vi "trafficLight.vi"() -> ()   [LabVIEW 2019]
uses:
  TrafficLight/control/Control 1.ctl
panel:
  in  "stop 2":bool
  in  "Process Stop Button":bool
  in  "green sec":i32
  in  "yellow sec":i32
  in  "red sec":i32
  out "red":bool
  out "yellow":bool
  out "green":bool
  out "秒數積累":i32
  in  "快走速度(ms)":u32=100
  in  "慢走速度(ms)":u32=200
  in  "轉速時間(S)":dbl=5.0
  out "Array":bool[][](array[boolean])=[[FALSE, FALSE, FALSE, FALSE, FALSE, FALSE, FALSE, FALSE, FALSE, FALSE, FALSE, FALSE, FALSE, FALSE, FALSE], [FALSE, FALSE, FALSE, FALSE, FALSE, FALSE, TRUE, TRUE, FALSE, FALSE, FALSE, FALSE, FALSE, FALSE, FALSE], [FALSE, FALSE, FALSE, FALSE, FALSE, TRUE, TRUE, TRUE, TRUE, FALSE, FALSE, FALSE, FALSE, FALSE, FALSE], [FALSE, FALSE, FALSE, FALSE, FALSE, TRUE, TRUE, TRUE, TRUE, FALSE, FALSE, FALSE, FALSE, FALSE, FALSE], [FALSE, FALSE, FALSE, FALSE, FALSE, FALSE, TRUE, TRUE, FALSE, FALSE, FALSE, FALSE, FALSE, FALSE, FALSE], [FALSE, FALSE, FALSE, FALSE, TRUE, TRUE, TRUE, TRUE, TRUE, TRUE, FALSE, FALSE, FALSE, FALSE, FALSE], [FALSE, FALSE, FALSE, TRUE, TRUE, TRUE, TRUE, TRUE, TRUE, TRUE, TRUE, FALSE, FALSE, FALSE, FALSE], [FALSE, FALSE, TRUE, TRUE, FALSE, TRUE, TRUE, TRUE, TRUE, FALSE, TRUE, TRUE, FALSE, FALSE, FALSE], [FALSE, FALSE, TRUE, TRUE, FALSE, TRUE, TRUE, TRUE, TRUE, FALSE, TRUE, TRUE, FALSE, FALSE, FALSE], [FALSE, FALSE, TRUE, FALSE, FALSE, TRUE, TRUE, TRUE, TRUE, FALSE, FALSE, TRUE, FALSE, FALSE, FALSE], [FALSE, FALSE, FALSE, FALSE, FALSE, TRUE, TRUE, TRUE, TRUE, FALSE, FALSE, FALSE, FALSE, FALSE, FALSE], [FALSE, FALSE, FALSE, FALSE, TRUE, TRUE, FALSE, FALSE, TRUE, TRUE, FALSE, FALSE, FALSE, FALSE, FALSE], [FALSE, FALSE, FALSE, FALSE, TRUE, TRUE, FALSE, FALSE, TRUE, TRUE, FALSE, FALSE, FALSE, FALSE, FALSE], [FALSE, FALSE, FALSE, TRUE, TRUE, FALSE, FALSE, FALSE, FALSE, TRUE, TRUE, FALSE, FALSE, FALSE, FALSE], [FALSE, FALSE, FALSE, TRUE, TRUE, FALSE, FALSE, FALSE, FALSE, TRUE, TRUE, FALSE, FALSE, FALSE, FALSE], [FALSE, FALSE, FALSE, TRUE, TRUE, FALSE, FALSE, FALSE, FALSE, TRUE, TRUE, FALSE, FALSE, FALSE, FALSE], [FALSE, FALSE, FALSE, FALSE, FALSE, FALSE, FALSE, FALSE, FALSE, FALSE, FALSE, FALSE, FALSE, FALSE, FALSE]]
  out "subarray":bool[][](array[boolean])
  in  "x-1":dbl
  out "剩餘時間 2":u32
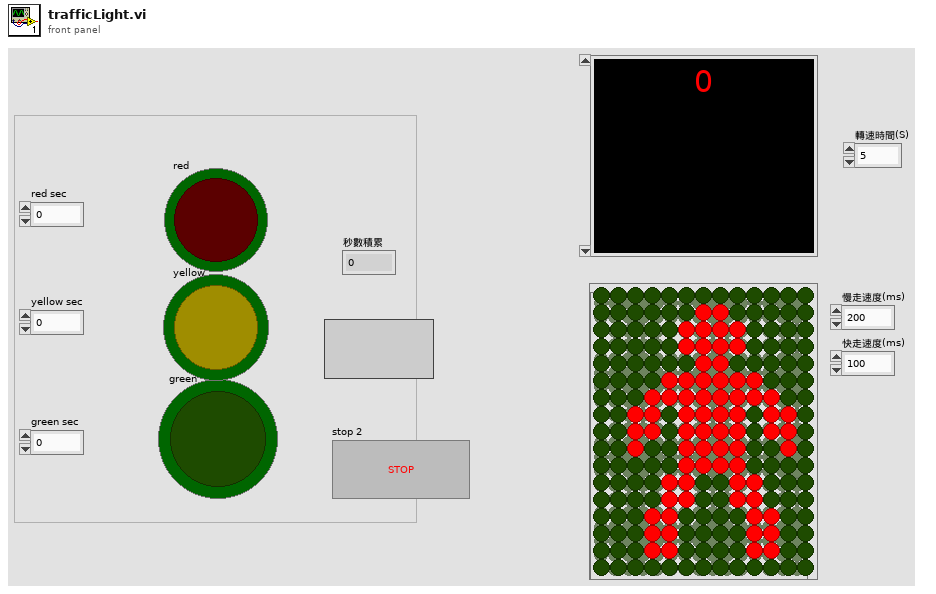
[diagram p1: front panel]
types:
  T1 = typedef "Control 1.ctl" = enum16{"red", "yellow", "green"}
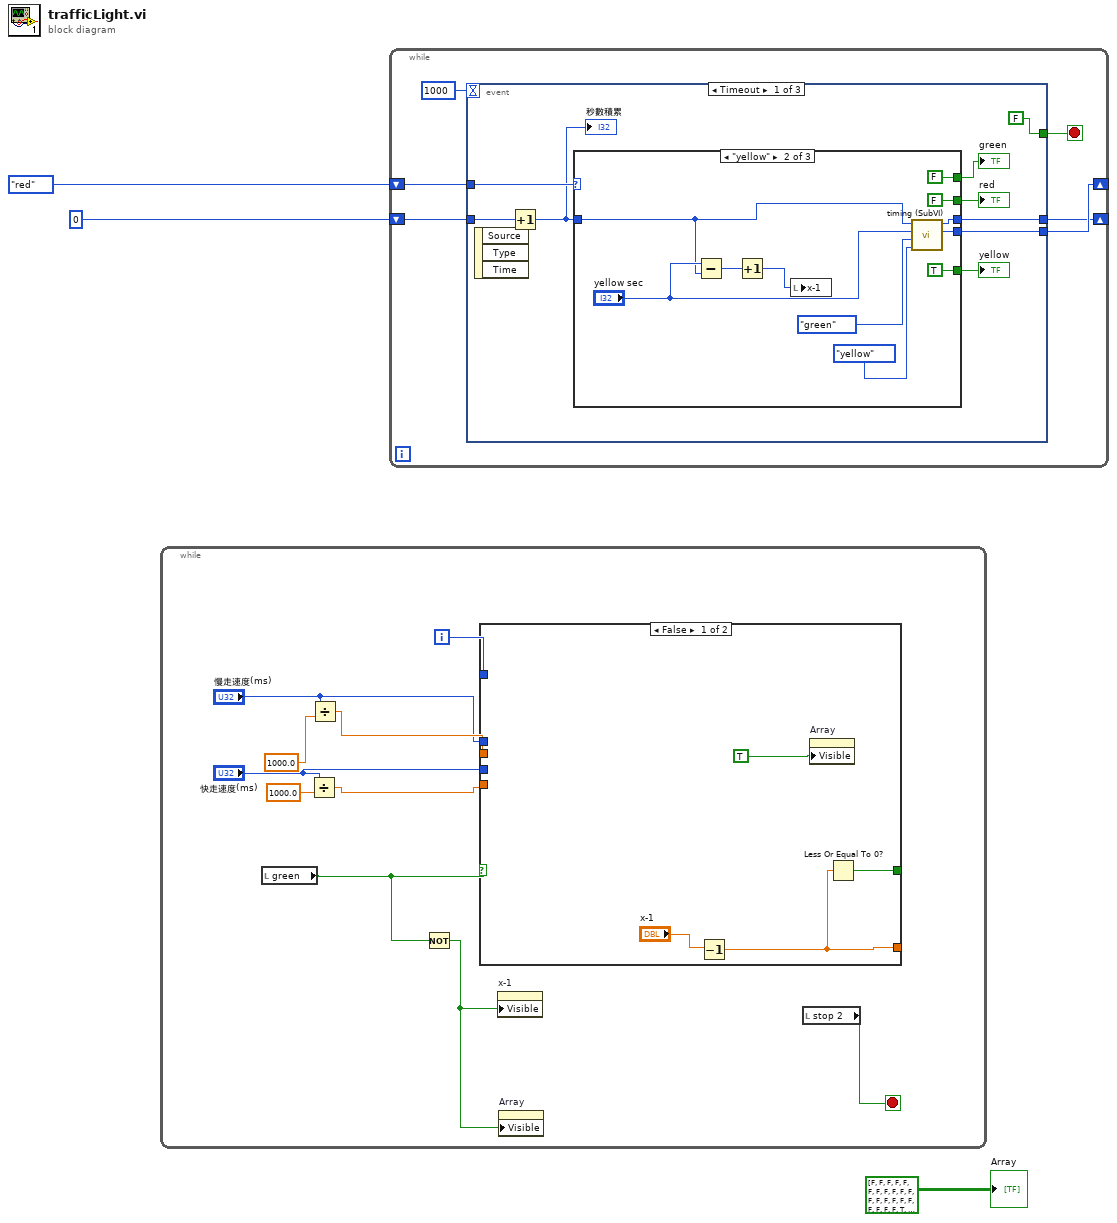
[diagram p0: block diagram]
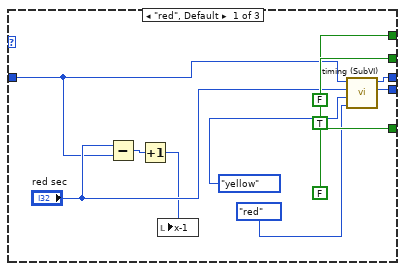
[diagram p2: hidden frame]
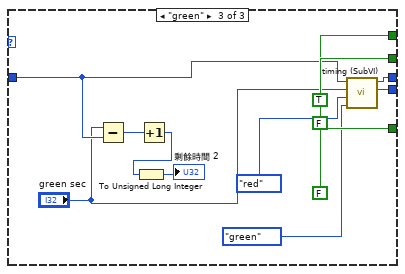
[diagram p3: hidden frame]
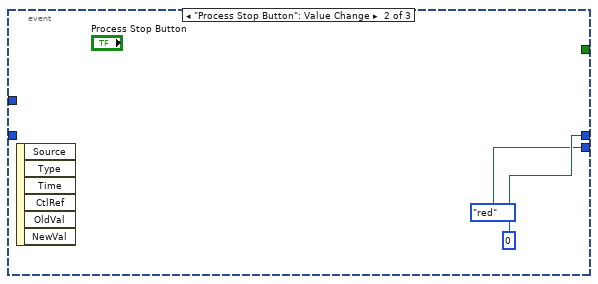
[diagram p4: hidden frame]
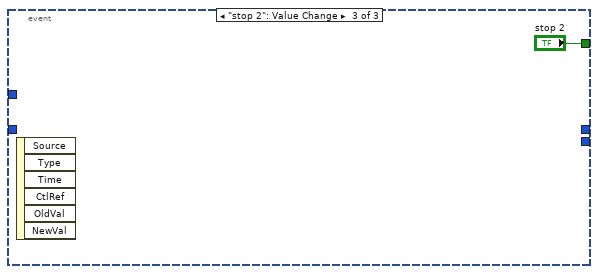
[diagram p5: hidden frame]
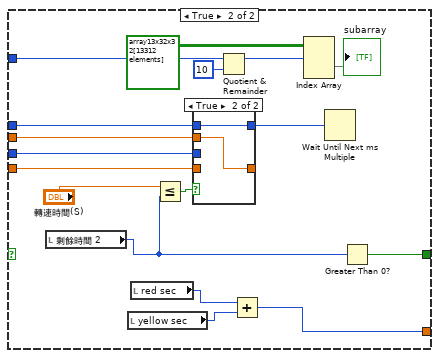
[diagram p6: hidden frame]
diagram:
  n1 = while {
    i -> [w12]
    stop <- w11 stop-if-true
    n2 = local read "green"() -> (w10:bool)
    n3 = Divide(x="快走速度(ms)", y=1000.0) -> (x/y=w6:dbl)
    n4 = Divide(x="慢走速度(ms)", y=1000.0) -> (x/y=w7:dbl)
    n5 = Not(x=w10) -> (.not. x?=w13:bool)
    n6 = case shown="False" w10 {
      tunnel: "慢走速度(ms)" -> [_ w33]
      tunnel: "快走速度(ms)" -> [_ w31]
      tunnel: w7 -> [_ w30]
      tunnel: w6 -> [_ w29]
      tunnel: [w16 w21] -> _
      tunnel: [w15 w28] -> _
      tunnel: w12 -> [_ w22]
      frame False {
        n7 = Decrement(x="x-1") -> (x-1=w16:dbl)
        n8 = property on="Array" class="Arr (strict)"("Visible"=TRUE) -> ()  [unwired: 2 in, 2 out]
        n9 = Less Or Equal To 0?(x=w16) -> (x <= 0?=w15:bool)
      }
      frame True {
        n10 = local read "剩餘時間 2"() -> (w18:u32)
        n11 = local read "yellow sec"() -> (w20:i32)
        n12 = local read "red sec"() -> (w19:i32)
        n13 = Less Or Equal?(x="轉速時間(S)", y=w18) -> (x <= y?=w34:bool)
        n14 = case shown="True" w34 {
          tunnel: w33 -> [_ w38]
          tunnel: [w36 w38] -> w32
          tunnel: w31 -> [w36 _]
          tunnel: w30 -> [_ w37]
          tunnel: [w35 w37] -> _
          tunnel: w29 -> [w35 _]
          frame False {
          }
          frame True {
          }
        }
        n15 = Quotient & Remainder(x=w22, y=10) -> (x-y*floor(x/y)=w25:i32)  [unwired: 1 out]
        n16 = Add(x=w19, y=w20) -> (x+y=w21:i32)
        n17 = Index Array(array=bool[][][] array13x32x32[13312 elements] ("小綠人1 2"), index (dim 0)=w25) -> (element=→"subarray":bool[][])  [unwired: 2 in]
        n18 = Wait Until Next ms Multiple(millisecond multiple=w32) -> ()  [unwired: 1 out]
        n19 = Greater Than 0?(x=w18) -> (x > 0?=w28:bool)
      }
    }
    n20 = property on="x-1" class="DigNum (strict)"("Visible"=w13) -> ()  [unwired: 2 in, 2 out]
    n21 = property on="Array" class="Arr (strict)"("Visible"=w13) -> ()  [unwired: 2 in, 2 out]
    n22 = local read "stop 2"() -> (w11:bool)
  }
  n23 = while {
    shift-right: [w43] -> _
    shift-left: Control_1."red" -> [w44]
    shift-right: [w41] -> _
    shift-left: 0 -> [w42]
    stop <- w39 stop-if-true
    n24 = event shown="[0] Timeout" {
      selector: _ -> [_ _ _]
      dyn-events: _ -> [_ _ _]
      timeout: u32 1000 ("milliseconds to wait") -> [_ _ _]
      tunnel: w44 -> [w53 _ _]
      tunnel: [w49 Control_1."red" _] -> w43
      tunnel: w42 -> [w48 _ _]
      tunnel: [w46 0 ("Numeric out") _] -> w41
      tunnel: [FALSE ("stop") _ "stop 2"] -> w39
      event Timeout {
        n25 = event-data() -> ()  [unwired: 1 in, 3 out]
        n26 = Increment(x=w48) -> (x+1=w47:i32)
        "秒數積累" <- w47
        n27 = case shown="\"yellow\"" w53 {
          tunnel: [TRUE FALSE FALSE] -> w52
          tunnel: [FALSE TRUE FALSE] -> w51
          tunnel: [FALSE FALSE TRUE] -> w50
          tunnel: [w61 w69 w81] -> w49
          tunnel: w47 -> [w55 w66 w80]
          tunnel: [w59 w70 w82] -> w46
          frame "red", Default {
            n28 = Subtract(x="red sec", y=w55) -> (x-y=w57:i32)
            n29 = Increment(x=w57) -> (x+1=w54:i32)
            n30 = local write "x-1"(w54) -> ()
            n31 = call "timing (SubVI).vi"("Enum F"=Control_1."red", "Enum T"=Control_1."yellow", "red sec"="red sec", "Numeric in"=w55) -> ("Enum out"=w61:T1, "Numeric out"=w59:i32)  [unwired: 6 in]
          }
          frame "yellow" {
            n32 = Subtract(x="yellow sec", y=w66) -> (x-y=w68:i32)
            n33 = Increment(x=w68) -> (x+1=w65:i32)
            n34 = local write "x-1"(w65) -> ()
            n35 = call "timing (SubVI).vi"("Enum F"=Control_1."yellow", "Enum T"=Control_1."green", "red sec"="yellow sec", "Numeric in"=w66) -> ("Enum out"=w69:T1, "Numeric out"=w70:i32)  [unwired: 6 in]
          }
          frame "green" {
            n36 = Subtract(x="green sec", y=w80) -> (x-y=w78:i32)
            n37 = Increment(x=w78) -> (x+1=w76:i32)
            n38 = To Unsigned Long Integer(number=w76) -> (unsigned 32bit integer=→"剩餘時間 2":u32)
            n39 = call "timing (SubVI).vi"("Enum F"=Control_1."green", "Enum T"=Control_1."red", "red sec"="green sec", "Numeric in"=w80) -> ("Enum out"=w81:T1, "Numeric out"=w82:i32)  [unwired: 6 in]
          }
        }
        "red" <- w52
        "yellow" <- w51
        "green" <- w50
      }
      event "Process Stop Button": Value Change {
        n40 = event-data() -> ()  [unwired: 1 in, 6 out]
      }
      event "stop 2": Value Change {
        n41 = event-data() -> ()  [unwired: 1 in, 6 out]
      }
    }
  }
  "Array" <- bool[][] [[FALSE, FALSE, FALSE, FALSE, FALSE, FALSE, FALSE, FALSE, FALSE, FALSE, FALSE, FALSE, FALSE, FALSE, FALSE], [FALSE, FALSE, FALSE, FALSE, FALSE, FALSE, TRUE, TRUE, FALSE, FALSE, FALSE, FALSE, FALSE, FALSE, FALSE], [FALSE, FALSE, FALSE, FALSE, FALSE, TRUE, TRUE, TRUE, TRUE, FALSE, FALSE, FALSE, FALSE, FALSE, FALSE], [FALSE, FALSE, FALSE, FALSE, FALSE, TRUE, TRUE, TRUE, TRUE, FALSE, FALSE, FALSE, FALSE, FALSE, FALSE], [FALSE, FALSE, FALSE, FALSE, FALSE, FALSE, TRUE, TRUE, FALSE, FALSE, FALSE, FALSE, FALSE, FALSE, FALSE], [FALSE, FALSE, FALSE, FALSE, TRUE, TRUE, TRUE, TRUE, TRUE, TRUE, FALSE, FALSE, FALSE, FALSE, FALSE], [FALSE, FALSE, FALSE, TRUE, TRUE, TRUE, TRUE, TRUE, TRUE, TRUE, TRUE, FALSE, FALSE, FALSE, FALSE], [FALSE, FALSE, TRUE, TRUE, FALSE, TRUE, TRUE, TRUE, TRUE, FALSE, TRUE, TRUE, FALSE, FALSE, FALSE], [FALSE, FALSE, TRUE, TRUE, FALSE, TRUE, TRUE, TRUE, TRUE, FALSE, TRUE, TRUE, FALSE, FALSE, FALSE], [FALSE, FALSE, TRUE, FALSE, FALSE, TRUE, TRUE, TRUE, TRUE, FALSE, FALSE, TRUE, FALSE, FALSE, FALSE], [FALSE, FALSE, FALSE, FALSE, FALSE, TRUE, TRUE, TRUE, TRUE, FALSE, FALSE, FALSE, FALSE, FALSE, FALSE], [FALSE, FALSE, FALSE, FALSE, TRUE, TRUE, FALSE, FALSE, TRUE, TRUE, FALSE, FALSE, FALSE, FALSE, FALSE], [FALSE, FALSE, FALSE, FALSE, TRUE, TRUE, FALSE, FALSE, TRUE, TRUE, FALSE, FALSE, FALSE, FALSE, FALSE], [FALSE, FALSE, FALSE, TRUE, TRUE, FALSE, FALSE, FALSE, FALSE, TRUE, TRUE, FALSE, FALSE, FALSE, FALSE], [FALSE, FALSE, FALSE, TRUE, TRUE, FALSE, FALSE, FALSE, FALSE, TRUE, TRUE, FALSE, FALSE, FALSE, FALSE], [FALSE, FALSE, FALSE, TRUE, TRUE, FALSE, FALSE, FALSE, FALSE, TRUE, TRUE, FALSE, FALSE, FALSE, FALSE], [FALSE, FALSE, FALSE, FALSE, FALSE, FALSE, FALSE, FALSE, FALSE, FALSE, FALSE, FALSE, FALSE, FALSE, FALSE]] ("Array")
